vi "Stop Core.vi"(10 "final error code":i32, 11 "Sim User Console Actor in":refnum<class "Sim User Console Actor.lvclass">) -> (3 "Sim User Console Actor out":refnum<class "Sim User Console Actor.lvclass">)   [LabVIEW 2022 SP3, in "Sim User Console Actor.lvlib" / "Sim User Console Actor.lvclass"]
doc: "(<B>Filename</B>: Actor Framework.lvlib:Actor.lvclass:Stop Core.vi)\n\nDefines what the actor does before it stops. Use the <B>final error code</B> input to determine whether the actor shut down in response to an error.\n\nBy default, this method does nothing. A descendant class may override it to define behavior, such as shutting down any processes the actor initiated in its override of the Actor Core method."
uses:
  Sim User Console Actor.lvclass
  Sim User Console Actor.lvclass/Sim User Console Actor.ctl
  Abstract User Console Actor/Abstract User Console Actor/Abstract User Console Actor.lvclass
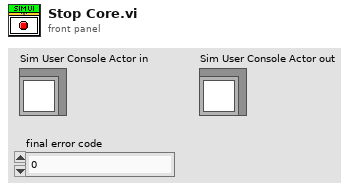
[diagram p1: front panel]
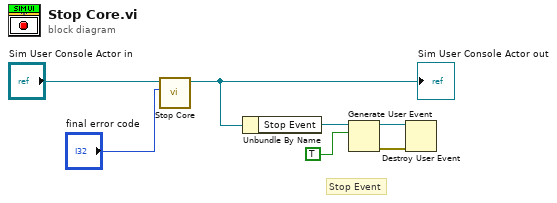
[diagram p0: block diagram]
diagram:
  # "Stop Event"
  n1 = call-parent "Stop Core.vi"("final error code"="final error code", "Actor in"="Sim User Console Actor in") -> ("Actor out"=w1:refnum<class "Sim User Console Actor.lvclass">)  [unwired: 9 in]
  "Sim User Console Actor out" <- w1
  n2 = Unbundle By Name(w1) -> ("Stop Event"=w2:refnum<user-event>)
  n3 = Generate User Event(user event=w2, event data cluster=TRUE ("event data")) -> (user event out=w4:refnum<user-event>, error out=w5:errorcluster)  [unwired: 2 in]
  n4 = Destroy User Event(user event=w4, error in=w5) -> ()  [unwired: 1 out]
